vi "FTW-File-UserDirectories.vi"(0 "Publisher (Organization)":string, 5 "Application (Product Name)":string) -> (4 "User Documents Dir":path, 6 "User Application Data Dir":path, 8 "User Preferences Dir":path, 10 "User Desktop":path)   [LabVIEW 2015]
panel:
  # "Inputs"
  # "Outputs"
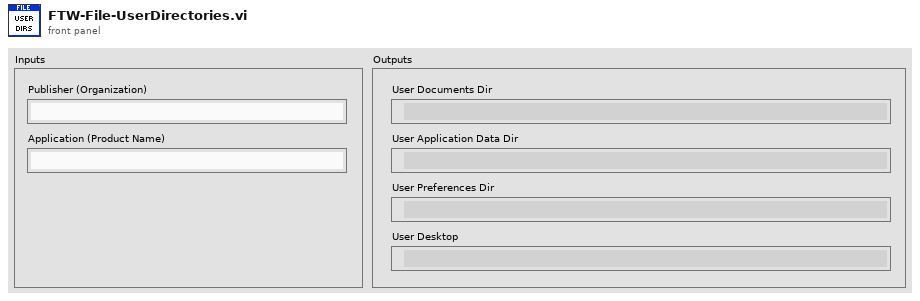
[diagram p1: front panel]
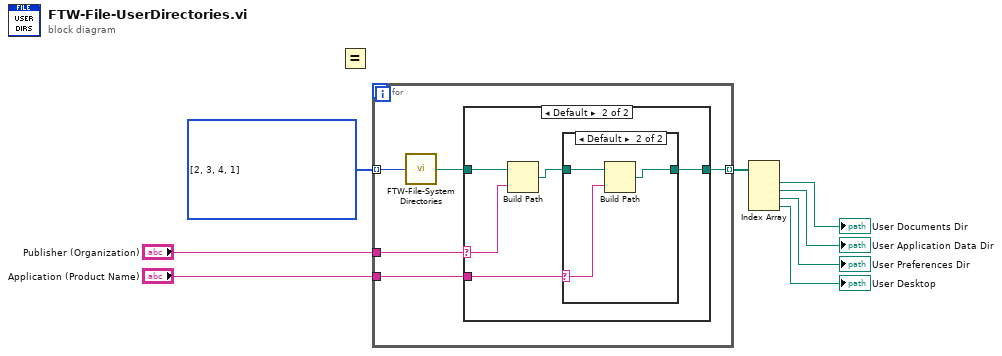
[diagram p0: block diagram]
diagram:
  w8 = i32[] [2, 3, 4, 1] items=["User Home"=0, "User Desktop"=1, "User Documents"=2, "User Application Data"=3, "User Preferences"=4, "User Temporary"=5, "Public Documents"=6, "Public Application Data"=7, "Public Preferences"=8, "Public Cache"=13, "System Core Libraries"=9, "System Installed Libraries"=10, "Application Files"=11, "Boot Volume Root"=12]
  n1 = Equal?() -> ()  [unwired: 2 in, 1 out]
  n2 = for {
    tunnel: w8 -> [w9] mode=indexing
    tunnel: "Application (Product Name)" -> [w13]
    tunnel: [w12] -> w6 mode=indexing
    tunnel: "Publisher (Organization)" -> [w11]
    n3 = call "FTW-File-SystemDirectories.vi"("System Directory"=w9) -> ("Directory"=w10:path)
    n4 = case shown="Default" w11 {
      selector: w11 -> [_ w15]
      tunnel: w10 -> [w14 w19]
      tunnel: w13 -> [_ w17]
      tunnel: [w14 w16] -> w12
      frame "" {
      }
      frame Default {
        n5 = Build Path(base path=w19, name or relative path=w15) -> (appended path=w18:path)
        n6 = case shown="Default" w17 {
          selector: w17 -> [_ w21]
          tunnel: w18 -> [w20 w23]
          tunnel: [w20 w22] -> w16
          frame "" {
          }
          frame Default {
            n7 = Build Path(base path=w23, name or relative path=w21) -> (appended path=w22:path)
          }
        }
      }
    }
  }
  n8 = Index Array(array=w6) -> (element #1=→"User Documents Dir":path, element #2=→"User Application Data Dir":path, element #3=→"User Preferences Dir":path, element #4=→"User Desktop":path)  [unwired: 4 in]
